vi "Write Scalar.vi"(8 "error in (no error)":errorcluster, 9 "Data":u8[](array[numeric]), 10 "Timestamp":u64, 11 "Ring buffer DVR in":refnum<data-value>) -> (0 "error out":errorcluster, 3 "Ring buffer DVR out":refnum<data-value>)   [LabVIEW 2021, in "Ring Buffer Time Series Data.lvlib"]
uses:
  Ring Buffer Time Series Data.lvlib
  SubVIs/DVR data.ctl
  SubVIs/Enforce array size one timestamp.vi
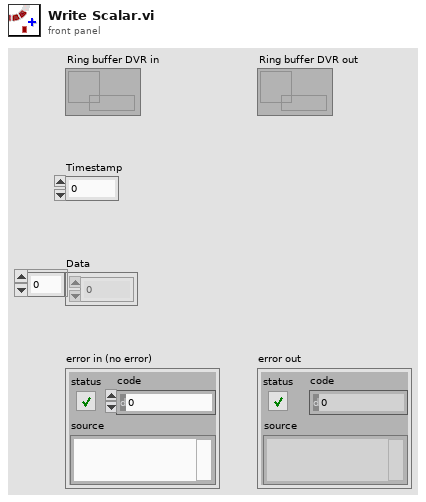
[diagram p1: front panel]
types:
  T1 = typedef "Ring Buffer Time Series Data.lvlib/DVR data.ctl" = cluster{"Timestamps":u64[], "Values":u8[], "#bytes per timestamp":i32, "Index":i32, "Size (#timestamps)":i32, "Full?":bool}
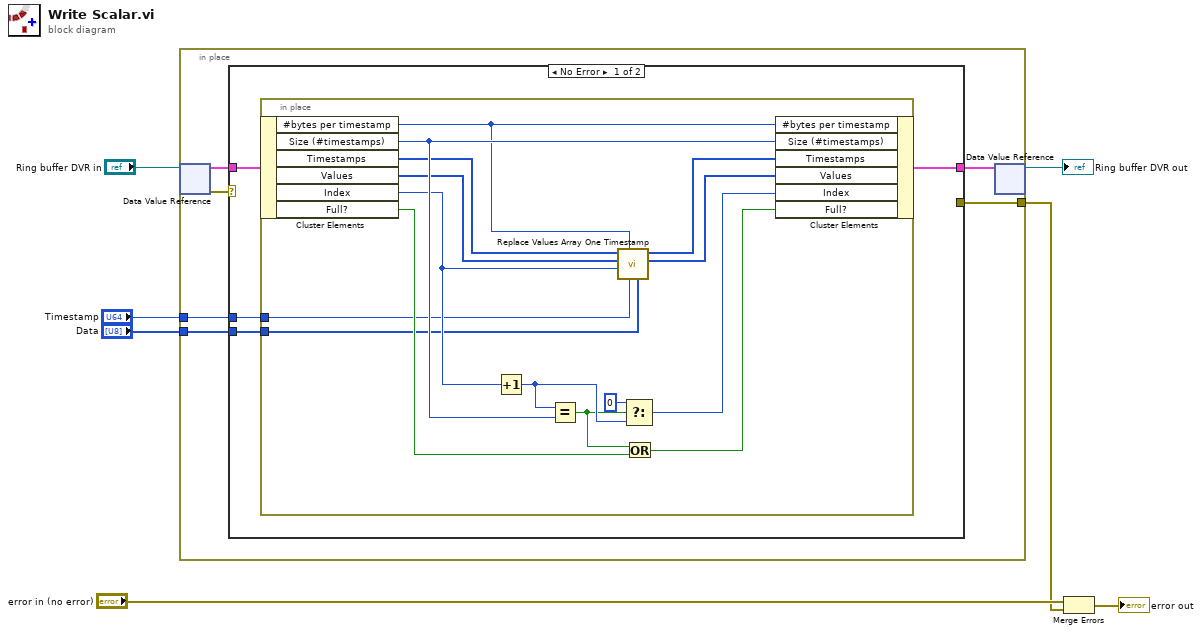
[diagram p0: block diagram]
diagram:
  n1 = in-place {
    in-place-border: [w10] -> w2
    in-place-border: "Timestamp" -> [w9]
    in-place-border: "Data" -> [w8]
    n2 = in-place-dvr #1("Ring buffer DVR in") -> (w12:T1, w13:errorcluster)
    n3 = case shown="No Error" w13 {
      selector: w13 -> [_ w33]
      tunnel: w12 -> [w17 _]
      tunnel: [w16 _] -> w11
      tunnel: [_ w33] -> w10
      tunnel: w9 -> [w15 _]
      tunnel: w8 -> [w14 _]
      frame No Error {
        n4 = in-place {
          in-place-border: w15 -> [w19]
          in-place-border: w14 -> [w18]
          n5 = in-place-cluster #2(w17) -> ("#bytes per timestamp"=w20:i32, "Size (#timestamps)"=w29:i32, "Timestamps"=w25:u64[], "Values"=w24:u8[], "Index"=w23:i32, "Full?"=w27:bool)
          n6 = Increment(x=w23) -> (x+1=w32:i32)
          n7 = Equal?(x=w32, y=w29) -> (x = y?=w28:bool)
          n8 = call "Replace Values Array One Timestamp.vi"("Values (new)"=w18, "Timestamps (new)"=w19, "#bytes per timestamp"=w20, "index"=w23, "Values (buffered)"=w24, "Timestamps (buffered)"=w25) -> ("Values (buffered)"=w21:u8[], "Timestamps (buffered)"=w22:u64[])  [unwired: 4 in]
          n9 = Select(t=0, s=w28, f=w32) -> (s? t:f=w30:i32)
          n10 = Or(x=w28, y=w27) -> (x .or. y?=w26:bool)
          n11 = in-place-cluster #2("#bytes per timestamp"=w20, "Size (#timestamps)"=w29, "Timestamps"=w22, "Values"=w21, "Index"=w30, "Full?"=w26) -> (w16:T1)
        }
      }
      frame Error {
      }
    }
    n12 = in-place-dvr #1(w11) -> (→"Ring buffer DVR out":refnum<data-value>)  [unwired: 1 out]
  }
  n13 = Merge Errors("error in (no error)", w2) -> (→"error out":errorcluster)
